vi "PAN_exe_system.vi"(7 "wait until completion? (T)":bool=TRUE, 8 "error in (no error)":errorcluster, 9 "command line":string, 10 "working directory":path=path "") -> (0 "error out":errorcluster, 2 "response":string)   [LabVIEW 2016]
uses:
  <vilib>/Utility/error.llb/DialogType.ctl
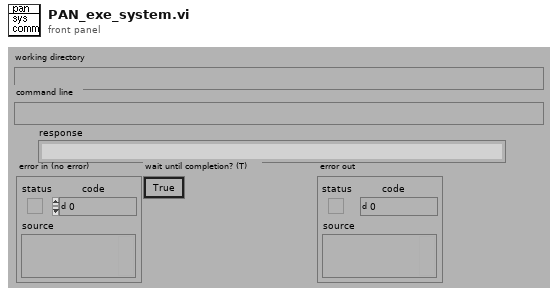
[diagram p1: front panel]
types:
  T1 = typedef "DialogType.ctl" = u16
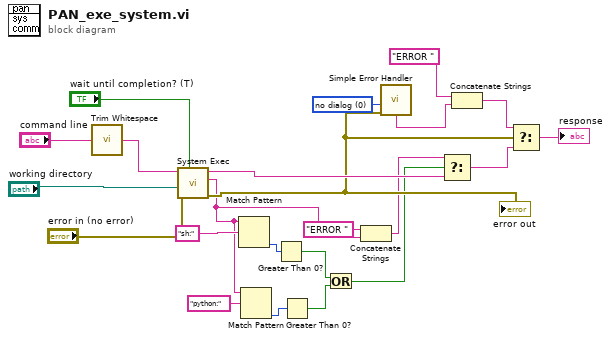
[diagram p0: block diagram]
diagram:
  w20 = T1 0 items=["no dialog", "OK message", "continue or stop message", "OK message + warnings", "continue/stop + warnings"] ("type of dialog (OK msg:1)")
  n1 = call <vilib>:"Trim Whitespace.vi"("string"="command line") -> ("trimmed string"=w3:string)  [unwired: 1 in]
  n2 = call <vilib>:"System Exec.vi"("wait until completion? (T)"="wait until completion? (T)", "error in (no error)"="error in (no error)", "working directory"="working directory", "command line"=w3) -> ("error out"=w19:errorcluster, "standard error"=w6:string, "standard output"=w23:string)  [unwired: 2 in, 3 out]
  "error out" <- w19
  n3 = Match Pattern(string=w6, regular expression="sh:") -> (offset past match=w16:i32)  [unwired: 4 out]
  n4 = Match Pattern(string=w6, regular expression="python:") -> (offset past match=w14:i32)  [unwired: 4 out]
  n5 = Greater Than 0?(x=w16) -> (x > 0?=w13:bool)
  n6 = Greater Than 0?(x=w14) -> (x > 0?=w12:bool)
  n7 = Or(x=w13, y=w12) -> (x .or. y?=w11:bool)
  n8 = Concatenate Strings("ERROR " ("string"), w6) -> (w5:string)
  n9 = call <vilib>:"Simple Error Handler.vi"("type of dialog (OK msg:1)"=w20, "error in (no error)"=w19) -> ("message"=w8:string)  [unwired: 7 out]
  n10 = Select(t=w5, s=w11, f=w23) -> (s? t:f=w10:string)
  n11 = Concatenate Strings("ERROR " ("string"), w8) -> (w7:string)
  n12 = Select(t=w7, s=w19, f=w10) -> (s? t:f=→"response":string)
